vi "APU + Knock Compile test.vi"() -> ()   [LabVIEW 2013]
uses:
  IP Source/APU/Settings.ctl
  IP Source/APU/Input.ctl
  IP Source/APU/Output.ctl
  IP Source/Knock Sensor/Generate Settings.ctl
  IP Source/Knock Sensor/Cylinder Settings.ctl
  IP Source/APU/Shared Settings.ctl
  IP Source/Knock Sensor/Cylinder Input.ctl
  IP Source/Version Token.ctl
  IP Source/Knock Sensor/Generate Input.ctl
  <vilib>/Platform/TimedLoop/XDataNode/timing_clust.ctl
  <vilib>/Platform/TimedLoop/XDataNode/nitl_modes.ctl
  <vilib>/Platform/TimedLoop/XDataNode/wakeup.ctl
  <vilib>/rvi/Emulation/niFpgaSctlEmulationGetInTimedLoop.vi
  <vilib>/rvi/Emulation/niFpgaEmulationReportErrorSimple.vi
  <vilib>/rvi/Emulation/niFpgaGetClockAttributes.vi
  <vilib>/rvi/Emulation/niFpgaCriticalErrorInLSC.vi
  <vilib>/rvi/eio/common/nirviEmuTemplateMethod_errors.vi
  <vilib>/Platform/TimedLoop/XDataNode/XDataNode.xnode
  <vilib>/eio/EIONode/EIONode.xnode
  <vilib>/Platform/TimedLoop/XDataNode/XDNodeRunTimeDep.lvlib
  IP Source/APU/APU.lvlib
  IP Source/Knock Sensor/Knock Sensor.lvlib
  IP Source/Engine Simulation Toolkit.lvlib
panel:
  in  "go.my apu":bool
  in  "input.Knock AO0":T1
  in  "est.version":T2
  in  "input.Knock AO0.Cylinder 4":T3
  in  "input.Knock AO0.Cylinder 3":T3
  in  "input.Knock AO0.Cylinder 2":T3
  in  "input.Knock AO0.Cylinder 1":T3
  in  "shared settings.my apu":T4 {"cycle start" format="%#.15g"}
  in  "settings.Knock AO0.Cylinder 4":T5
  in  "settings.Knock AO0.Cylinder 3":T5
  in  "settings.Knock AO0.Cylinder 2":T5
  in  "settings.Knock AO0.Cylinder 1":T5
  in  "settings.Knock AO0":T6
  out "output.my apu":T7 caption="output"
  in  "input.my apu":T8={"desired speed"=0.0, "reset"=TRUE} caption="input"
  in  "settings.my apu":T9 caption="settings"
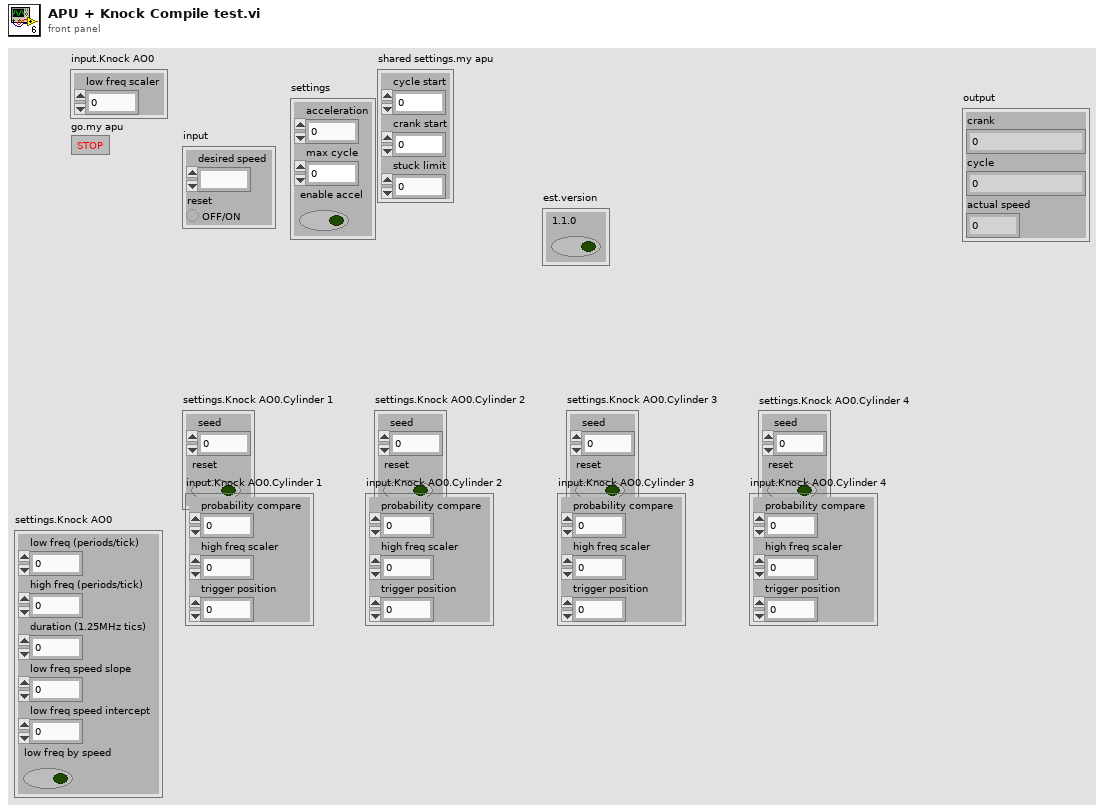
[diagram p1: front panel]
types:
  T1 = typedef "Engine Simulation Toolkit.lvlib/Knock Sensor.lvlib/Generate Input.ctl" = cluster{"low freq scaler":fxp<+,10,0>}
  T2 = typedef "Engine Simulation Toolkit.lvlib/Version Token.ctl" = cluster{"1.1.0":bool}
  T3 = typedef "Engine Simulation Toolkit.lvlib/Knock Sensor.lvlib/Cylinder Input.ctl" = cluster{"probability compare":u16, "high freq scaler":fxp<+,10,0>, "trigger position":u16}
  T4 = typedef "Engine Simulation Toolkit.lvlib/APU.lvlib/Shared Settings.ctl" = cluster{"cycle start":fxp<+,2,2>, "crank start":u16, "stuck limit":fxp<+,18,18>}
  T5 = typedef "Engine Simulation Toolkit.lvlib/Knock Sensor.lvlib/Cylinder Settings.ctl" = cluster{"seed":u16, "reset":bool}
  T6 = typedef "Engine Simulation Toolkit.lvlib/Knock Sensor.lvlib/Generate Settings.ctl" = cluster{"low freq (periods/tick)":fxp<+,32,0>, "high freq (periods/tick)":fxp<+,32,0>, "duration (1.25MHz tics)":fxp<+,18,18>, "low freq speed slope":fxp<+,16,-3>, "low freq speed intercept":fxp<+,10,-10>, "low freq by speed":bool}
  T7 = typedef "Engine Simulation Toolkit.lvlib/APU.lvlib/Output.ctl" = cluster{"crank":u16, "cycle":u16, "actual speed":fxp<+/-,23,2>}
  T8 = typedef "Engine Simulation Toolkit.lvlib/APU.lvlib/Input.ctl" = cluster{"desired speed":fxp<+/-,23,2>, "reset":bool}
  T9 = typedef "Engine Simulation Toolkit.lvlib/APU.lvlib/Settings.ctl" = cluster{"acceleration":fxp<+,18,-20>, "max cycle":fxp<+,2,2>, "enable accel":bool}
  T10 = typedef "XDNodeRunTimeDep.lvlib/timing_clust.ctl" = cluster{"Expected End [f-1]":u64, "Actual End [f-1]":u64, "Finished Late? [f-1]":bool, "Expected End [i-1]":u64, "Actual End [i-1]":u64, "Finished Late? [i-1]":bool, "Expected Start [i]":u64, "Actual Start [i]":u64, "Expected Start [f]":u64, "Actual Start [f]":u64, "Source Name":string, "Structure Name":string, "Period":i64, "Deadline":i64, "Offset":i64, "Start":i64, "Priority":i32, "Timeout":i32, "Mode":T11, "Wakeup Reason":T12, "Error":errorcluster, "Source Type":string, "Secondary Source Type":string, "Global End Time":u64, "Global Start Time":u64, "Frame Duration":u64, "Iteration Duration":u64, "Assigned CPU":i32, "I/O Scan Engine Mode":u32}
  T11 = typedef "XDNodeRunTimeDep.lvlib/nitl_modes.ctl" = enum32{"No Change", "Process missed periods, maintain original phase", "Discard missed periods, maintain original phase", "Process missed periods, ignore original phase", "Discard missed periods, ignore original phase"}
  T12 = typedef "XDNodeRunTimeDep.lvlib/wakeup.ctl" = enum32{"Normal", "Aborted", "Asynchronous wakeup", "Timing source error", "Timed loop error", "Timeout"}
  T13 = typedef "Engine Simulation Toolkit.lvlib/APU.lvlib/Register Bus.ctl" = cluster{"Speed":refnum<k21>, "Crank Angle":refnum<k21>, "Cycle Angle":refnum<k21>, "Crank Count":refnum<k21>, "Cycle Count":refnum<k21>, "1.25 MHz Counter":refnum<k21>, "shared settings":T4}
  T14 = typedef "Engine Simulation Toolkit.lvlib/Knock Sensor.lvlib/Triggered Cylinder Data.ctl" = cluster{"trigger knock":bool, "high freq scaler":fxp<+,10,0>}
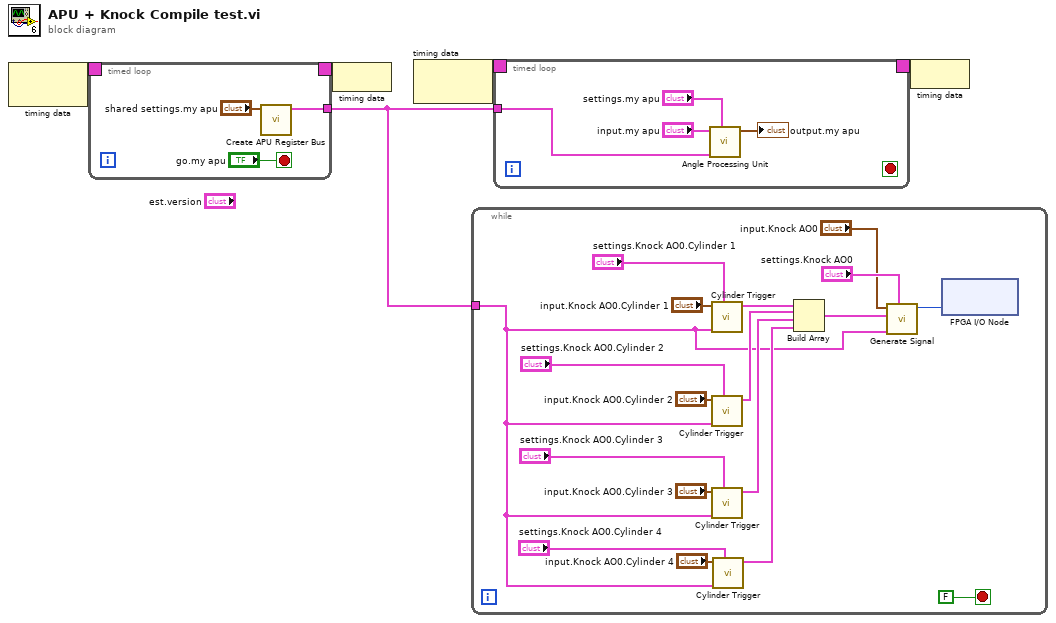
[diagram p0: block diagram]
diagram:
  n1 = node-c288() -> (w2:T10)  [unwired: 1 in]
  n2 = timed-loop {
    timing: w2 -> [_]
    timing-out: [_] -> w1
    tunnel: [w8] -> w3
    stop <- "go.my apu" stop-if-true
    n3 = call "Create APU Register Bus.vi"("shared settings.<user name>"="shared settings.my apu") -> ("register bus"=w8:T13)  [unwired: 10 in]
  }
  n4 = node-c288(w1) -> ()
  n5 = node-c288() -> (w5:T10)  [unwired: 1 in]
  n6 = while {
    tunnel: w3 -> [w13]
    stop <- FALSE stop-if-true
    n7 = call "Cylinder Trigger.vi"("settings.<user name>"="settings.Knock AO0.Cylinder 1", "register bus"=w13, "input.<user name>"="input.Knock AO0.Cylinder 1") -> ("triggered knock data"=w28:T14)  [unwired: 8 in]
    n8 = call "Cylinder Trigger.vi"("settings.<user name>"="settings.Knock AO0.Cylinder 2", "register bus"=w13, "input.<user name>"="input.Knock AO0.Cylinder 2") -> ("triggered knock data"=w27:T14)  [unwired: 8 in]
    n9 = call "Cylinder Trigger.vi"("settings.<user name>"="settings.Knock AO0.Cylinder 3", "register bus"=w13, "input.<user name>"="input.Knock AO0.Cylinder 3") -> ("triggered knock data"=w26:T14)  [unwired: 8 in]
    n10 = call "Cylinder Trigger.vi"("settings.<user name>"="settings.Knock AO0.Cylinder 4", "register bus"=w13, "input.<user name>"="input.Knock AO0.Cylinder 4") -> ("triggered knock data"=w25:T14)  [unwired: 8 in]
    n11 = Build Array(w28, w27, w26, w25) -> (w24:T14[])
    n12 = call "Generate Signal.vi"("settings.<user name>"="settings.Knock AO0", "register bus"=w13, "triggered knock data"=w24, "input.<user name>"="input.Knock AO0") -> ("knock signal"=w14:i16)  [unwired: 7 in]
    n13 = xnode "FPGA I/O Node"("AO0"=w14) -> ()  [unwired: 1 in, 1 out]
  }
  n14 = timed-loop {
    timing: w5 -> [_]
    timing-out: [_] -> w4
    tunnel: w3 -> [w29]
    stop <- _ stop-if-true
    n15 = call "Angle Processing Unit.vi"("settings.<user name>"="settings.my apu", "register bus"=w29, "input.<user name>"="input.my apu") -> ("output.<user name>"=→"output.my apu":T7)  [unwired: 8 in]
  }
  n16 = node-c288(w4) -> ()
